vi "IconIsSet.vi"(9 "expected":T1, 10 "icon":T1) -> (0 "error out":errorcluster)   [LabVIEW 2017, in "ResultTree.Tests.lvlib" / "SetIcon.lvlib"]
uses:
  SetIcon.lvlib
  ResultTree/Icon.ctl
  c545755b-2565-431d-95b3-e7ded266f0f0.vi
  Constraint/IsEqual/Create.vi
  Constraint/IsEqual/IsEqual.lvclass
  ResultTree/ResultTree.lvclass
panel:
  in  "Tree":string(tree)
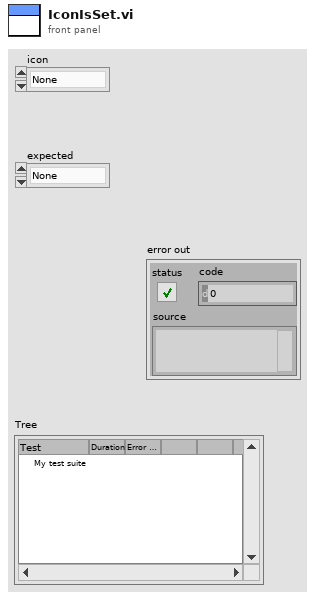
[diagram p1: front panel]
types:
  T1 = typedef "ResultTree.lvclass/Icon.ctl" = enum16{"None", "Passed", "Failed", "Error"}
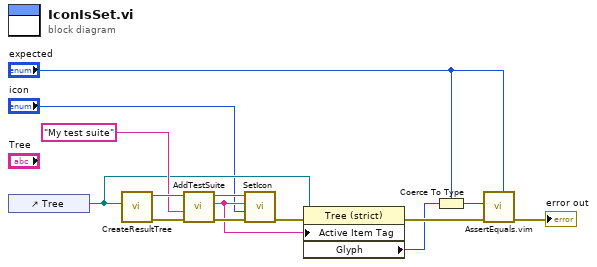
[diagram p0: block diagram]
diagram:
  n1 = control-ref of="Tree"() -> (w8:refnum<vi>)
  n2 = call "CreateResultTree.vi"("Tree Refnum"=w8) -> ("error out"=w13:errorcluster, "ResultTree out"=w12:refnum<class "ResultTree.lvclass">)  [unwired: 9 in]
  n3 = call "AddTestSuite.vi"("error in (no error)"=w13, "Name"="My test suite", "ResultTree in"=w12) -> ("error out"=w10:errorcluster, "Tag Name"=w5:string, "ResultTree out"=w9:refnum<class "ResultTree.lvclass">)  [unwired: 6 in]
  n4 = call "SetIcon.vi"("error in (no error)"=w10, "Icon"="icon", "Tag Name"=w5, "ResultTree in"=w9) -> ("error out"=w7:errorcluster)  [unwired: 6 in, 1 out]
  n5 = property class="Tree (strict)"(reference=w8, error in=w7, "Active Item Tag"=w5) -> (error out=w6:errorcluster, "Glyph"=w4:i32)  [unwired: 1 out]
  n6 = Coerce To Type(0:w4, 1:"expected") -> (2:w2:T1)
  n7 = call "AssertEquals.vim"("Expected"="expected", "error in (no error)"=w6, "Actual"=w2) -> ("error out"=→"error out":errorcluster)  [unwired: 8 in]
